vi "FGV_ConnectionProperties.vi"(7 "Enum":T1, 8 "Frontend Status in":string, 9 "Connection Attempt in":u32, 10 "MIDAS Port in":u16, 11 "MIDAS Addresss in":string) -> (0 "Frontend Status out":string, 1 "Connection Attempt out":u32, 2 "MIDAS Port out":u16, 3 "MIDAS Addresss out":string)   [LabVIEW 2018, in "feGEM DataPacker.lvlib"]
uses:
  Set_And_Get_Enum.ctl
  feGEM DataPacker.lvlib
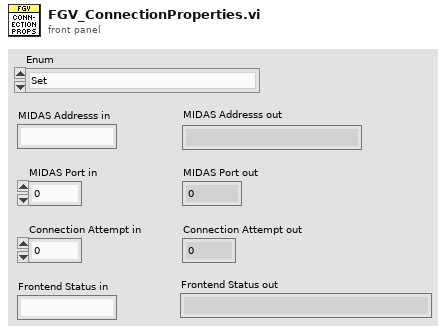
[diagram p1: front panel]
types:
  T1 = typedef "feGEM DataPacker.lvlib/Set_And_Get_Enum.ctl" = enum16{"Set", "Get"}
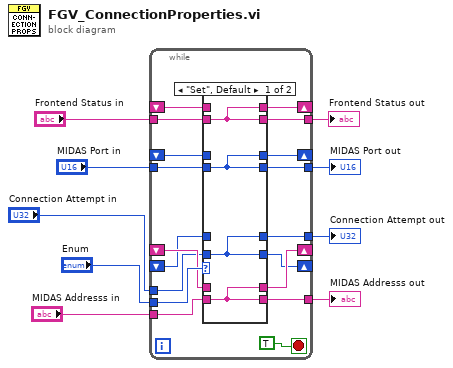
[diagram p0: block diagram]
diagram:
  n1 = while {
    tunnel: "MIDAS Addresss in" -> [w25]
    tunnel: "Enum" -> [w27]
    tunnel: [w24] -> w7
    shift-right: [w23] -> _
    shift-left: _ -> [w22]
    tunnel: "MIDAS Port in" -> [w21]
    tunnel: [w20] -> w5
    shift-right: [w19] -> _
    shift-left: _ -> [w18]
    tunnel: "Connection Attempt in" -> [w17]
    tunnel: [w16] -> w3
    shift-right: [w15] -> _
    shift-left: _ -> [w14]
    tunnel: "Frontend Status in" -> [w13]
    tunnel: [w12] -> w1
    shift-right: [w11] -> _
    shift-left: _ -> [w10]
    stop <- TRUE stop-if-true
    n2 = case shown="\"Set\", Default" w27 {
      tunnel: w25 -> [w31 _]
      tunnel: [w31 w35] -> w24
      tunnel: [w31 w35] -> w23
      tunnel: w22 -> [_ w35]
      tunnel: w21 -> [w30 _]
      tunnel: [w30 w34] -> w20
      tunnel: [w30 w34] -> w19
      tunnel: w18 -> [_ w34]
      tunnel: w17 -> [w29 _]
      tunnel: [w29 w33] -> w16
      tunnel: [w29 w33] -> w15
      tunnel: w14 -> [_ w33]
      tunnel: w13 -> [w28 _]
      tunnel: [w28 w32] -> w12
      tunnel: [w28 w32] -> w11
      tunnel: w10 -> [_ w32]
      frame "Set", Default {
      }
      frame "Get" {
      }
    }
  }
  "Frontend Status out" <- w1
  "MIDAS Port out" <- w5
  "MIDAS Addresss out" <- w7
  "Connection Attempt out" <- w3
